vi "Module.Gui.Translate.vi"(8 "error in":errorcluster, 10 "flag?":bool, 11 "VI ref in":refnum<vi>) -> (0 "error out":errorcluster, 2 "language flag":picture, 3 "VI ref out":refnum<vi>)   [LabVIEW 2019, in "Tools.lvlib"]
uses:
  Tools.lvlib
  TMOS config/TMOS.Config.Action.ctl
  ProjectPaths.ctl
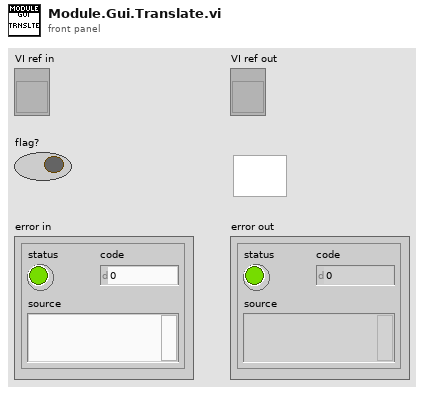
[diagram p1: front panel]
types:
  T1 = typedef "TMOS.Config.Action.ctl" = enum16{"init", "update", "get", "set"}
  T2 = typedef "Tools.lvlib/ProjectPaths.ctl" = enum16{"Settings dir", "Logs dir", "Resources dir", "Verification file", "Users file", "Root dir"}
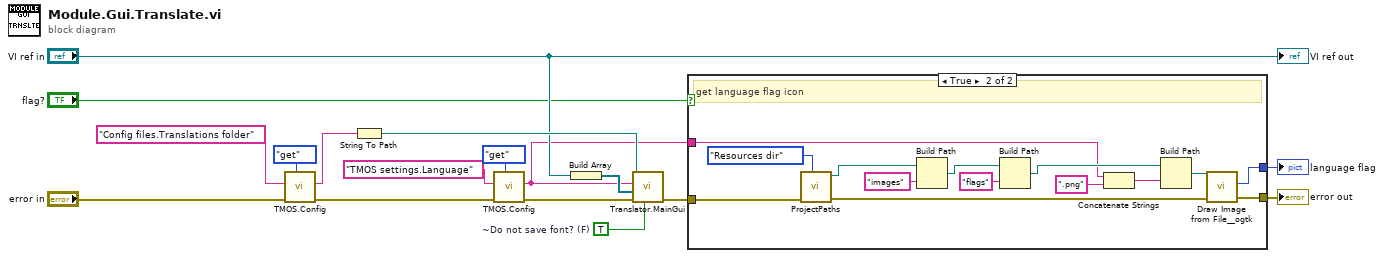
[diagram p0: block diagram]
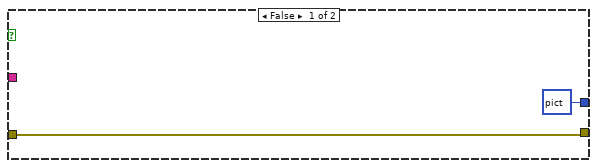
[diagram p2: hidden frame]
diagram:
  w2 = TRUE  # ~Do not save font? (F)
  n1 = call "TMOS.Config.vi"("action"=TMOS.Config.Action."get", "error in"="error in", "name"="Config files.Translations folder" ("~Language in use")) -> ("error out"=w13:errorcluster, "read value"=w16:string)  [unwired: 6 in, 1 out]
  n2 = String To Path(string=w16) -> (path=w17:path)
  n3 = call "TMOS.Config.vi"("action"=TMOS.Config.Action."get", "error in"=w13, "name"="TMOS settings.Language" ("~Language in use")) -> ("error out"=w9:errorcluster, "read value"=w1:string)  [unwired: 6 in, 1 out]
  n4 = Build Array("VI ref in") -> (w3:refnum<vi>[])
  n5 = call "Translator.MainGui.vi"("~Do not save font? (F)"=w2, "~error in"=w9, "VI ref in [ ]"=w3, "~Language in use"=w1, "~Translation folder"=w17) -> ("~error out"=w6:errorcluster)  [unwired: 3 in, 3 out]
  n6 = case shown="True" "flag?" {
    tunnel: [picture data[5B] ("new picture") w33] -> w7
    tunnel: w1 -> [_ w24]
    tunnel: w6 -> [w19 w22]
    tunnel: [w19 w21] -> w5
    frame False {
    }
    frame True {
      # "get language flag icon"
      n7 = call "ProjectPaths.vi"("Item"=ProjectPaths."Resources dir", "Error In"=w22) -> ("Error Out"=w23:errorcluster, "Path"=w32:path)  [unwired: 8 in]
      n8 = Build Path(base path=w32, name or relative path="images") -> (appended path=w30:path)
      n9 = Build Path(base path=w30, name or relative path="flags") -> (appended path=w28:path)
      n10 = Concatenate Strings(w24, ".png" ("string")) -> (w27:string)
      n11 = Build Path(base path=w28, name or relative path=w27) -> (appended path=w25:path)
      n12 = call <userlib>:"Draw Image from File__ogtk.vi"("error in (no error)"=w23, "path to image file"=w25) -> ("error out"=w21:errorcluster, "new picture"=w33:picture)  [unwired: 6 in, 2 out]
    }
  }
  "error out" <- w5
  "language flag" <- w7
  "VI ref out" <- "VI ref in"
